vi "Write StimulationPK.vi"(8 "error in (no error)":errorcluster, 10 "StimulationPK":T1, 11 "TrialBasedExperiment in":refnum<class "TrialBasedExperiment.lvclass">) -> (0 "error out":errorcluster, 3 "TrialBasedExperiment out":refnum<class "TrialBasedExperiment.lvclass">)   [LabVIEW 2014, in "AcquisitionCoreObjects.lvlib" / "TrialBasedExperiment.lvclass"]
uses:
  TrialBasedExperiment.lvclass
  Acquisition/Database/StimulationPrimary.ctl
  TrialBasedExperiment.lvclass/TrialBasedExperiment.ctl
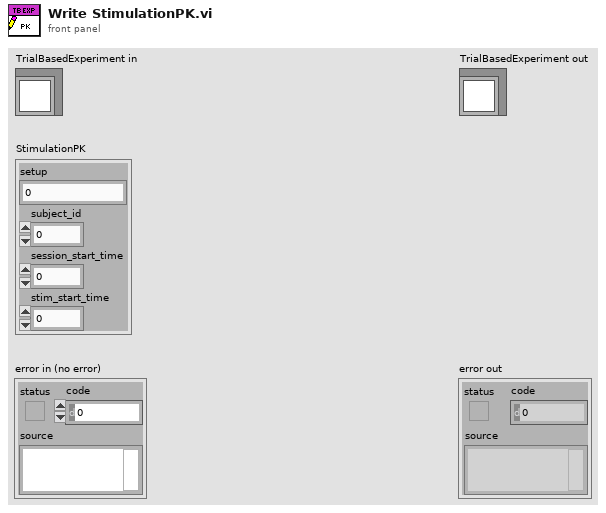
[diagram p1: front panel]
types:
  T1 = typedef "StimulationPrimary.ctl" = cluster{"setup":u8, "subject_id":i32, "session_start_time":dbl, "stim_start_time":dbl}
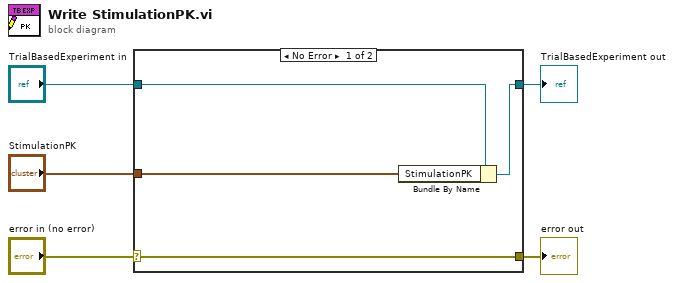
[diagram p0: block diagram]
diagram:
  n1 = case shown="No Error" "error in (no error)" {
    selector: "error in (no error)" -> [w9 w10]
    tunnel: [w9 w10] -> w4
    tunnel: [w7 w11] -> w2
    tunnel: "TrialBasedExperiment in" -> [w8 w11]
    tunnel: "StimulationPK" -> [w6 _]
    frame No Error {
      n2 = Bundle By Name(cluster=w8, "StimulationPK"=w6) -> (w7:refnum<class "TrialBasedExperiment.lvclass">)
    }
    frame Error {
    }
  }
  "error out" <- w4
  "TrialBasedExperiment out" <- w2
